vi "LWXPS_PositionerCorrectorDualGet.vi"(0 "XPS Reference IN":refnum<k24>, 2 "Positioner Name":string, 5 "LabVIEW error IN":errorcluster) -> (7 "LabVIEW error OUT":errorcluster, 8 "XPS Reference OUT":refnum<k24>, 9 "XPS Error String":string, 10 "Returned error code":i32, 11 "Anti wind up time":dbl, 12 "Closed Loop Status":bool, 13 "Jerk feedforward gain":dbl, 14 "Proportional gain":dbl, 15 "Integral gain":dbl, 16 "Derivative gain":dbl, 17 "Integration time":dbl, 18 "Derivative filter cut off frequency":dbl, 19 "Acceleration feedforward gain":dbl)   [LabVIEW 2014]
uses:
  D:/XPSQ8_LabView_Library/Development/Source/Dll/Newport.XPS.CommandInterface.dll
  Dll/Newport.XPS.CommandInterface.dll
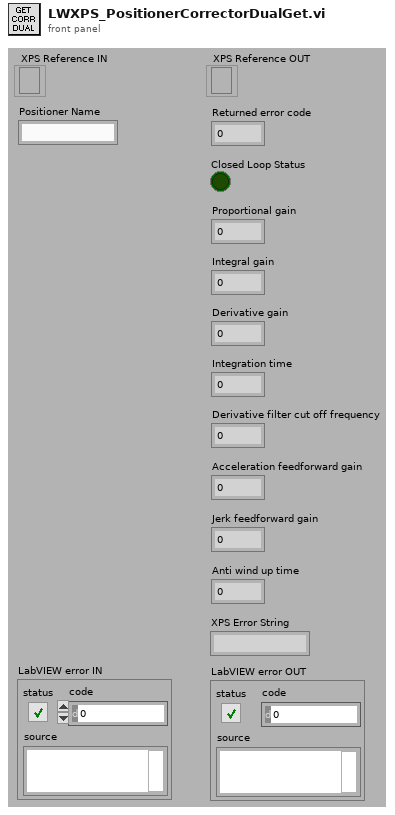
[diagram p1: front panel]
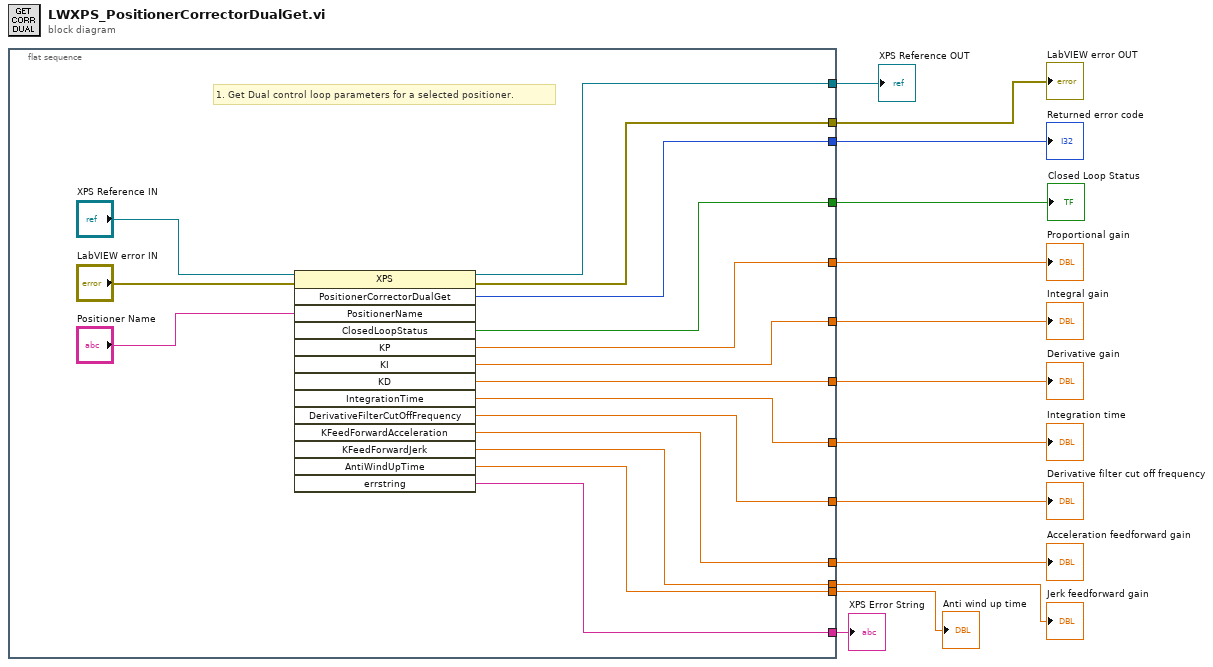
[diagram p0: block diagram]
diagram:
  n1 = flat-sequence {
    tunnel: [w27] -> w13
    tunnel: [w14] -> w12
    tunnel: [w28] -> w11
    tunnel: [w20] -> w1
    tunnel: [w23] -> w10
    tunnel: [w24] -> w7
    tunnel: [w22] -> w9
    tunnel: [w21] -> w8
    tunnel: [w19] -> w6
    tunnel: [w18] -> w5
    tunnel: [w17] -> w4
    tunnel: [w16] -> w3
    tunnel: [w15] -> w2
    frame #0 {
      # "1. Get Dual control loop parameters for a selected positioner."
      n2 = invoke class="XPS" method="PositionerCorrectorDualGet"(reference="XPS Reference IN", error in="LabVIEW error IN", "PositionerName"="Positioner Name") -> (reference out=w27:refnum<k24>, error out=w14:errorcluster, "PositionerCorrectorDualGet"=w28:i32, "ClosedLoopStatus"=w20:bool, "KP"=w23:dbl, "KI"=w22:dbl, "KD"=w21:dbl, "IntegrationTime"=w24:dbl, "DerivativeFilterCutOffFrequency"=w19:dbl, "KFeedForwardAcceleration"=w18:dbl, "KFeedForwardJerk"=w17:dbl, "AntiWindUpTime"=w16:dbl, "errstring"=w15:string)  [unwired: 11 in, 1 out]
    }
  }
  "XPS Error String" <- w2
  "XPS Reference OUT" <- w13
  "LabVIEW error OUT" <- w12
  "Returned error code" <- w11
  "Proportional gain" <- w10
  "Integral gain" <- w9
  "Derivative gain" <- w8
  "Integration time" <- w7
  "Derivative filter cut off frequency" <- w6
  "Acceleration feedforward gain" <- w5
  "Jerk feedforward gain" <- w4
  "Anti wind up time" <- w3
  "Closed Loop Status" <- w1
